vi "read_write.vi"(5 "Query?":bool, 6 "error in":errorcluster, 7 "Bytes to read":i32=1, 8 "Command":string, 9 "VISA handle in":refnum<visa-resource-name>) -> (0 "error out":errorcluster, 2 "Response":string, 3 "VISA handle out":refnum<visa-resource-name>, 4 "TimeoutFlag":bool)   [LabVIEW 2018]
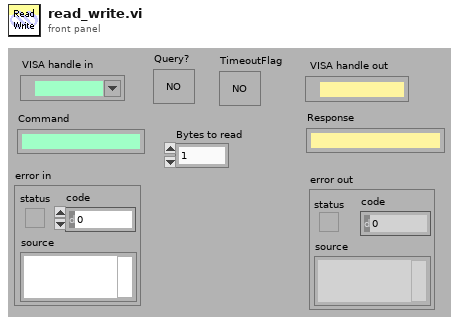
[diagram p1: front panel]
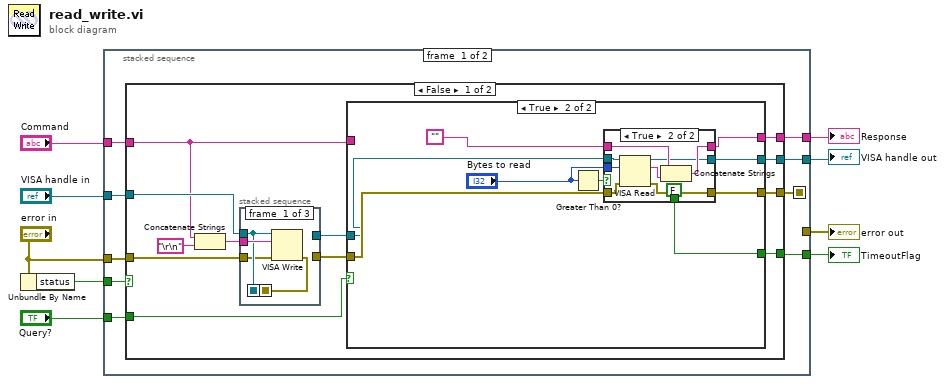
[diagram p0: block diagram]
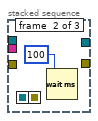
[diagram p2: hidden frame]
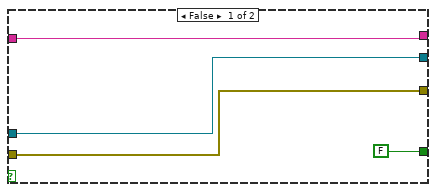
[diagram p4: hidden frame]
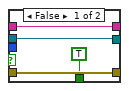
[diagram p5: hidden frame]
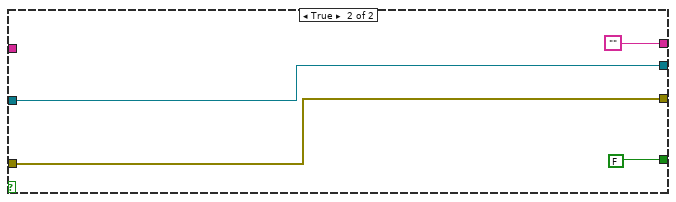
[diagram p6: hidden frame]
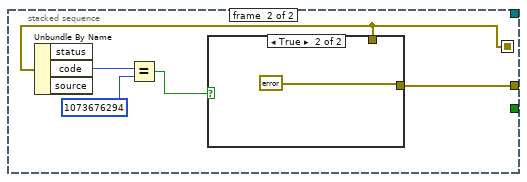
[diagram p7: hidden frame]
diagram:
  n1 = Unbundle By Name("error in") -> ("status"=w7:bool)
  n2 = stacked-sequence {
    seq-local: [w14 _] -> [_ w68]
    tunnel: "VISA handle in" -> [w18 _]
    tunnel: [_ w69] -> w8
    tunnel: w7 -> [w17 _]
    tunnel: "error in" -> [w16 _]
    tunnel: "Query?" -> [w15 _]
    tunnel: "Command" -> [w13 _]
    tunnel: [w12 _] -> w1
    tunnel: [w11 _] -> w3
    tunnel: [w10 _] -> w2
    frame #0 {
      n3 = case shown="False" w17 {
        tunnel: w18 -> [w30 w67]
        tunnel: [w26 w67] -> w12
        tunnel: [w25 w66] -> w14
        tunnel: w16 -> [w29 w66]
        tunnel: [w24 ""] -> w10
        tunnel: [w23 FALSE] -> w11
        tunnel: w15 -> [w20 _]
        tunnel: w13 -> [w19 _]
        frame False {
          n4 = Concatenate Strings(w19, "\r\n") -> (w21:string)
          n5 = stacked-sequence {
            seq-local: [w33 _ _] -> [_ _ w37]
            seq-local: [w31 _ _] -> [_ _ w36]
            tunnel: w30 -> [w33 _ _]
            tunnel: w21 -> [w34 _ _]
            tunnel: w29 -> [w32 _ _]
            tunnel: [_ _ w37] -> w28
            tunnel: [_ _ w36] -> w27
            frame #0 {
              n6 = VISA Write(VISA resource name=w33, write buffer=w34, error in (no error)=w32) -> (error out=w31:errorcluster)  [unwired: 2 out]
            }
            frame #1 {
              n7 = Wait (ms)(milliseconds to wait=u32 100 ("Delay (ms)")) -> ()  [unwired: 1 out]
            }
            frame #2 {
            }
          }
          n8 = case shown="True" w20 {
            tunnel: [w40 w47] -> w25
            tunnel: [w41 w50] -> w26
            tunnel: w28 -> [w41 w43]
            tunnel: w27 -> [w40 w44]
            tunnel: [w38 w49] -> w24
            tunnel: [FALSE w42] -> w23
            tunnel: w19 -> [w38 _]
            frame False {
            }
            frame True {
              n9 = Greater Than 0?(x="Bytes to read") -> (x > 0?=w46:bool)
              n10 = case shown="True" w46 {
                tunnel: "Bytes to read" -> [_ w63]
                tunnel: "" -> [w54 w61]
                tunnel: [w54 w60] -> w49
                tunnel: [w52 w59] -> w50
                tunnel: w44 -> [w53 w58]
                tunnel: [w53 w57] -> w47
                tunnel: w43 -> [w52 w56]
                tunnel: [TRUE FALSE] -> w42
                frame False {
                }
                frame True {
                  n11 = VISA Read(VISA resource name=w56, byte count=w63, error in (no error)=w58) -> (VISA resource name out=w59:refnum<visa-resource-name>, read buffer=w62:string, error out=w57:errorcluster)  [unwired: 1 out]
                  n12 = Concatenate Strings(w61, w62) -> (w60:string)
                }
              }
            }
          }
        }
        frame True {
        }
      }
    }
    frame #1 {
      n13 = Unbundle By Name(w68) -> ("code"=w72:i32)  [unwired: 2 out]
      n14 = Equal?(x=w72, y=1073676294) -> (x = y?=w71:bool)
      n15 = case shown="True" w71 {
        tunnel: w68 -> [w73 _]
        tunnel: [w73 errorcluster {"status"=FALSE, "code"=0, "source"=""} ("sortie d'erreur 2")] -> w69
        frame False {
        }
        frame True {
        }
      }
    }
  }
  "VISA handle out" <- w1
  "error out" <- w8
  "Response" <- w2
  "TimeoutFlag" <- w3
